vi "move_to_zero.vi"(8 "error in (no error)":errorcluster, 11 "VISA Refnum in":refnum<visa-resource-name>) -> (0 "error out":errorcluster, 3 "VISA resource name out":refnum<visa-resource-name>)   [LabVIEW 2014]
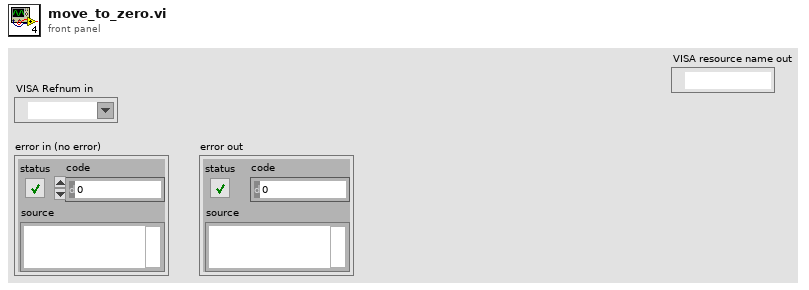
[diagram p1: front panel]
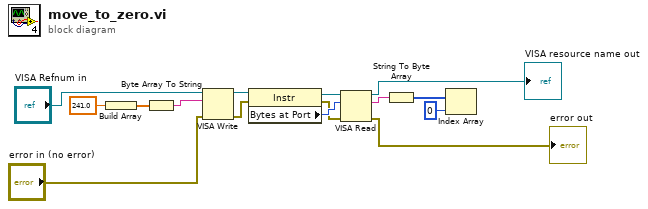
[diagram p0: block diagram]
diagram:
  n1 = Build Array(241.0 ("element")) -> (w7:dbl[])
  n2 = Byte Array To String(unsigned byte array=w7) -> (string=w6:string)
  n3 = VISA Write(VISA resource name="VISA Refnum in", write buffer=w6, error in (no error)="error in (no error)") -> (VISA resource name out=w8:refnum<visa-resource-name>, error out=w9:errorcluster)  [unwired: 1 out]
  n4 = property class="Instr"(reference=w8, error in=w9) -> (reference out=w13:refnum<visa-resource-name>, error out=w14:errorcluster, "Bytes at Port"=w15:u32)
  n5 = VISA Read(VISA resource name=w13, byte count=w15, error in (no error)=w14) -> (VISA resource name out=→"VISA resource name out":refnum<visa-resource-name>, read buffer=w4:string, error out=→"error out":errorcluster)  [unwired: 1 out]
  n6 = String To Byte Array(string=w4) -> (unsigned byte array=w2:u8[])
  n7 = Index Array(array=w2, index=0) -> ()  [unwired: 1 out]
